vi "Button_number.vi"(1 "Button Array":bool[](array[boolean])) -> (0 "Button Pressed":i32)   [LabVIEW 2013]
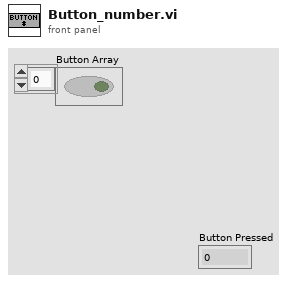
[diagram p1: front panel]
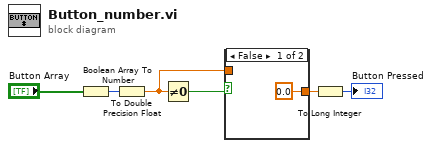
[diagram p0: block diagram]
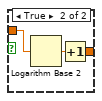
[diagram p2: hidden frame]
diagram:
  n1 = Boolean Array To Number(Boolean array="Button Array") -> (number=w6:u32)
  n2 = To Double Precision Float(number=w6) -> (double precision float=w3:dbl)
  n3 = Not Equal To 0?(x=w3) -> (x != 0?=w4:bool)
  n4 = case shown="False" w4 {
    tunnel: [0.0 w8] -> w5
    tunnel: w3 -> [_ w9]
    frame False {
    }
    frame True {
      n5 = Logarithm Base 2(1:w9) -> (0:w10:dbl)
      n6 = Increment(x=w10) -> (x+1=w8:dbl)
    }
  }
  n7 = To Long Integer(number=w5) -> (32bit integer=→"Button Pressed":i32)
